vi "Create Resources.vi"(11 "AO in":refnum<class "Analog Output.lvclass">) -> (2 "AO out":refnum<class "Analog Output.lvclass">, 3 "AO subsystem":refnum<class "Single Address Space Collection.lvclass">)   [LabVIEW 2017, in "Analog IO.lvlib" / "Analog Output.lvclass"]
uses:
  Analog Output.lvclass
  C:/Program Files (x86)/National Instruments/LabVIEW 2017/instr.lib/_niInstr/Instruction Framework/v1/FPGA/Interfaces/Address Space/Address Space.lvclass
  <instrlib>/_niInstr/Instruction Framework/v1/FPGA/Helper Classes/Single Address Space Collection/Single Address Space Collection.lvclass
  <instrlib>/_niInstr/Instruction Framework/v1/FPGA/Interfaces/Address Space/Address Space.lvclass
  Analog Output.lvclass/Analog Output.ctl
  <vilib>/rvi/DataTransferAndStorage/Container/Common/niFpgaContainerGetUniqueNameForEmu.vi
  <vilib>/rvi/DataTransferAndStorage/Container/Common/niFpgaContainerSetEmuInfo.vi
  <vilib>/rvi/eio/common/nirviEmuReportErrorAndStop.vi
  <vilib>/rvi/LocalResourceManager/LocalResourceManager.xnode
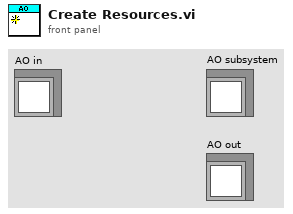
[diagram p1: front panel]
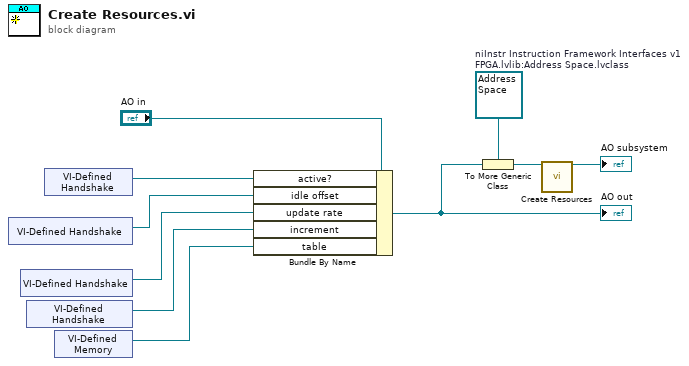
[diagram p0: block diagram]
diagram:
  w10 = refnum<class "Address Space.lvclass"> refnum  # niInstr Instruction Framework Interfaces v1 FPGA.lvlib:Address Space.lvclass
  n1 = xnode "VI-Defined Handshake"() -> ("Handshake Out"=w9:refnum<k21>)
  n2 = xnode "VI-Defined Handshake"() -> ("Handshake Out"=w3:refnum<k21>)
  n3 = xnode "VI-Defined Handshake"() -> ("Handshake Out"=w5:refnum<k21>)
  n4 = xnode "VI-Defined Handshake"() -> ("Handshake Out"=w1:refnum<k21>)
  n5 = xnode "VI-Defined Memory"() -> ("Memory Out"=w4:refnum<k21>)
  n6 = Bundle By Name(cluster="AO in", "active?"=w1, "idle offset"=w9, "update rate"=w3, "increment"=w5, "table"=w4) -> (w6:refnum<class "Analog Output.lvclass">)
  "AO out" <- w6
  n7 = To More Generic Class(target class=w10, reference=w6) -> (generic class reference=w8:refnum<class "Address Space.lvclass">)
  n8 = call "Create Resources.vi"("address space"=w8) -> ("single address space collection"=→"AO subsystem":refnum<class "Single Address Space Collection.lvclass">)  [unwired: 14 in]
